vi "Test TCRS Restarting Heating.vi"(8 "error in (no error)":errorcluster, 11 "Thermal Chamber Response Simlator Test In":refnum<class "Thermal Chamber Response Simlator Test.lvclass">) -> (0 "error out":errorcluster, 3 "Thermal Chamber Response Simlator Test Out":refnum<class "Thermal Chamber Response Simlator Test.lvclass">)   [LabVIEW 2020, in "Thermal Chamber Response Simlator Test.lvclass"]
uses:
  Thermal Chamber Response Simlator Test.lvclass
  Thermal Chamber Response Simlator/Thermal Chamber Response Simlator.lvclass
  <vilib>/Asteme/LUnit/Test Case.lvclass
  C:/Program Files (x86)/National Instruments/LabVIEW 2020/vi.lib/Asteme/LUnit/Test Case.lvclass
  C:/Users/anton/Documents/GitHub/Triarc-Examples/Thermal Chamber/Thermal Chamber Response Simlator Test/Thermal Chamber Response Simlator Test.lvclass
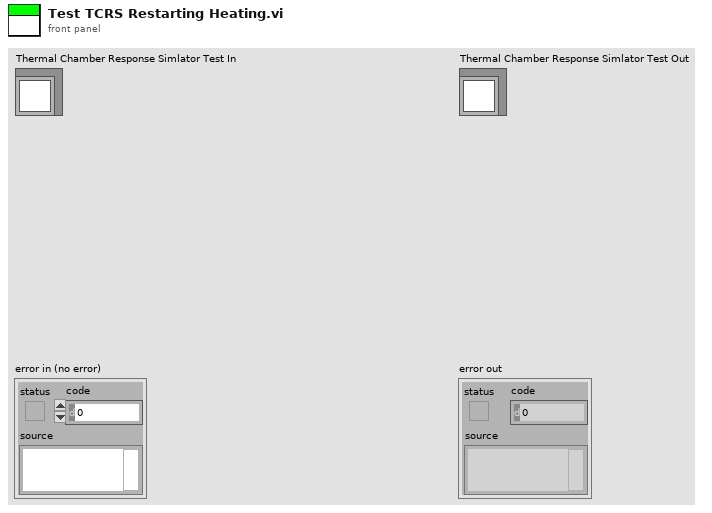
[diagram p1: front panel]
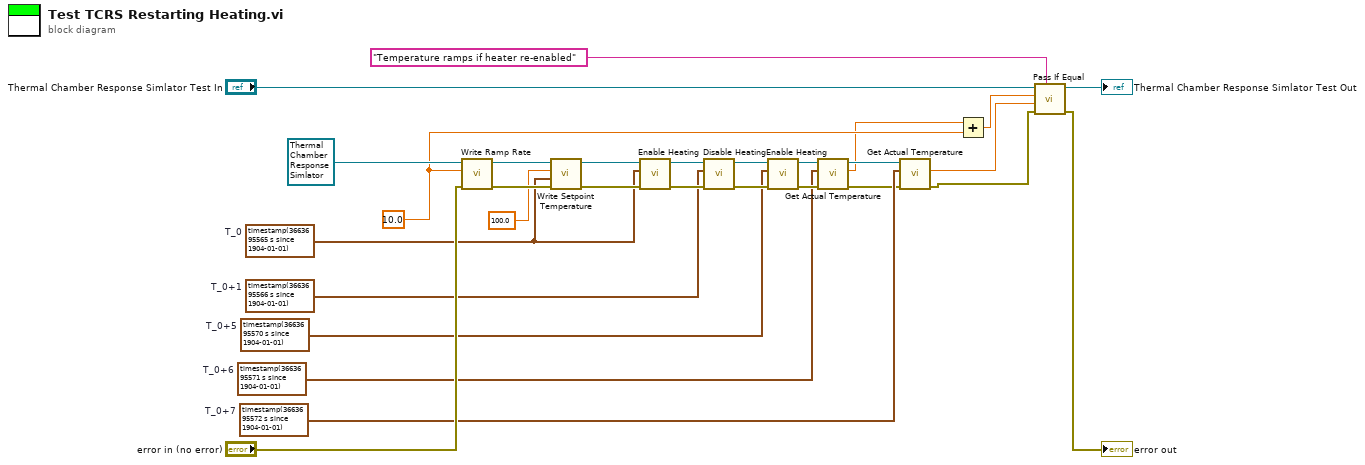
[diagram p0: block diagram]
diagram:
  w6 = timestamp(3663695572 s since 1904-01-01)  # T_0+7
  w13 = timestamp(3663695571 s since 1904-01-01)  # T_0+6
  w16 = timestamp(3663695570 s since 1904-01-01)  # T_0+5
  w17 = timestamp(3663695566 s since 1904-01-01)  # T_0+1
  w14 = 10.0 ("Ramp Rate [degC/s]")
  w8 = timestamp(3663695565 s since 1904-01-01)  # T_0
  n1 = call "Write Ramp Rate.vi"("error in (no error)"="error in (no error)", "Ramp Rate [degC/s]"=w14, "Thermal Chamber Response Simlator In"=refnum<class "Thermal Chamber Response Simlator.lvclass"> refnum ("Thermal Chamber Response Simlator.lvclass")) -> ("error out"=w28:errorcluster, "Thermal Chamber Response Simlator Out"=w11:refnum<class "Thermal Chamber Response Simlator.lvclass">)  [unwired: 7 in]
  n2 = call "Write Setpoint Temperature.vi"("error in (no error)"=w28, "Update Time"=w8, "Setpoint Temperature [degC]"=100.0, "Thermal Chamber Response Simlator In"=w11) -> ("error out"=w12:errorcluster, "Thermal Chamber Response Simlator Out"=w10:refnum<class "Thermal Chamber Response Simlator.lvclass">)  [unwired: 6 in]
  n3 = call "Enable Heating.vi"("error in (no error)"=w12, "Start Time"=w8, "Thermal Chamber Response Simlator In"=w10) -> ("error out"=w22:errorcluster, "Thermal Chamber Response Simlator Out"=w23:refnum<class "Thermal Chamber Response Simlator.lvclass">)  [unwired: 7 in]
  n4 = call "Disable Heating.vi"("error in (no error)"=w22, "Start Time"=w17, "Thermal Chamber Response Simlator In"=w23) -> ("error out"=w21:errorcluster, "Thermal Chamber Response Simlator Out"=w19:refnum<class "Thermal Chamber Response Simlator.lvclass">)  [unwired: 7 in]
  n5 = call "Enable Heating.vi"("error in (no error)"=w21, "Start Time"=w16, "Thermal Chamber Response Simlator In"=w19) -> ("error out"=w20:errorcluster, "Thermal Chamber Response Simlator Out"=w18:refnum<class "Thermal Chamber Response Simlator.lvclass">)  [unwired: 7 in]
  n6 = call "Get Actual Temperature.vi"("error in (no error)"=w20, "Time Stamp"=w13, "Thermal Chamber Response Simlator In"=w18) -> ("error out"=w5:errorcluster, "Actual Temperature [degC]"=w1:dbl, "Thermal Chamber Response Simlator Out"=w7:refnum<class "Thermal Chamber Response Simlator.lvclass">)  [unwired: 6 in]
  n7 = call "Get Actual Temperature.vi"("error in (no error)"=w5, "Time Stamp"=w6, "Thermal Chamber Response Simlator In"=w7) -> ("error out"=w3:errorcluster, "Actual Temperature [degC]"=w4:dbl)  [unwired: 6 in, 1 out]
  n8 = Add(x=w1, y=w14) -> (x+y=w15:dbl)
  n9 = call <vilib>:"Pass If Equal.vi"("Description"="Temperature ramps if heater re-enabled", "error in (no error)"=w3, "Actual"=w4, "Expected"=w15, "Test Case In"="Thermal Chamber Response Simlator Test In") -> ("error out"=→"error out":errorcluster, "Test Case Out"=→"Thermal Chamber Response Simlator Test Out":refnum<class "Thermal Chamber Response Simlator Test.lvclass">)  [unwired: 5 in]
